vi "Basic interface (lab view).vi"() -> ()   [LabVIEW 2019]
panel:
  out "Tangent":dbl
  out "Cosine":dbl
  out "Sine":dbl
  out "Radians 2":dbl
  in  "Degrees 2":dbl
  out "Radians":dbl
  in  "Degrees":dbl
  out "Degrees":dbl
  in  "Radians":dbl
  # "Radians to degrees"
  # "Degrees to Radians"
  # "Trignometric values for the given angle"
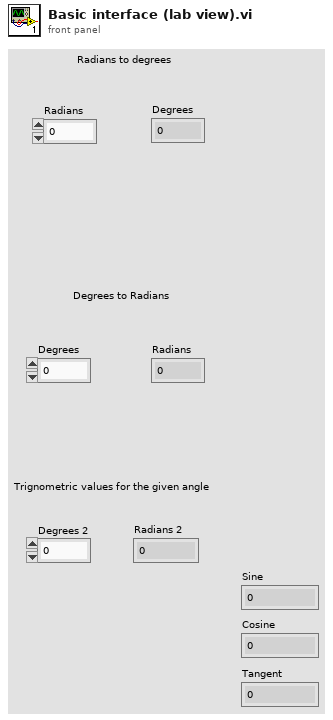
[diagram p1: front panel]
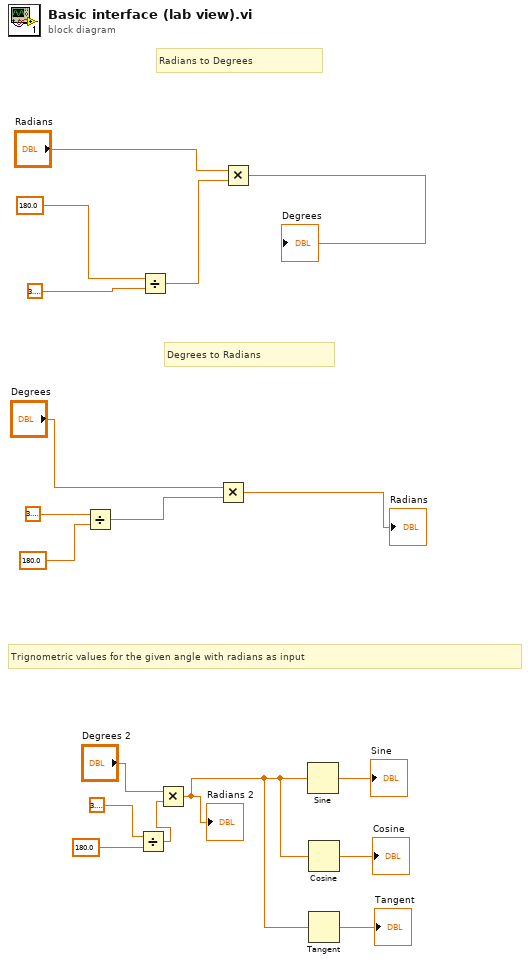
[diagram p0: block diagram]
diagram:
  # "Trignometric values for the given angle with radians as input"
  # "Degrees to Radians"
  # "Radians to Degrees"
  n1 = Divide(x=3.141592653589793, y=180.0) -> (x/y=w10:dbl)
  n2 = Divide(x=3.141592653589793, y=180.0) -> (x/y=w5:dbl)
  n3 = Divide(x=180.0, y=3.141592653589793) -> (x/y=w15:dbl)
  n4 = Multiply(x="Degrees 2", y=w5) -> (x*y=w3:dbl)
  "Radians 2" <- w3
  n5 = Multiply(x="Degrees", y=w10) -> (x*y=→"Radians":dbl)
  n6 = Multiply(x="Radians", y=w15) -> (x*y=→"Degrees":dbl)
  n7 = Sine(x=w3) -> (sin(x)=→"Sine":dbl)
  n8 = Cosine(x=w3) -> (cos(x)=→"Cosine":dbl)
  n9 = Tangent(1:w3) -> (0:→"Tangent":dbl)
